vi "ReadRingConstant.vi"(1 "reference":refnum<vi>) -> (0 "RingConstant":T6)   [LabVIEW 2013]
uses:
  <vilib>/Utility/miscctls.llb/LVBoundsTypeDef.ctl
  <vilib>/Utility/miscctls.llb/LVPositionTypeDef.ctl
  <vilib>/Utility/miscctls.llb/LVRectTypeDef.ctl
  <vilib>/numeric/LVNumericRepresentation.ctl
  <vilib>/Utility/miscctls.llb/LVStringsAndValuesArrayTypeDef.ctl
panel:
  out "error out 29":errorcluster
  out "error out 28":errorcluster
  out "error out 27":errorcluster
  out "error out 26":errorcluster
  out "error out 25":errorcluster
  out "error out 24":errorcluster
  out "error out 23":errorcluster
  out "error out 22":errorcluster
  out "error out 21":errorcluster
  out "error out 20":errorcluster
  out "error out 19":errorcluster
  out "error out 18":errorcluster
  out "error out 17":errorcluster
  out "error out 16":errorcluster
  out "error out 15":errorcluster
  out "error out 14":errorcluster
  out "error out 13":errorcluster
  out "error out 12":errorcluster
  out "error out 11":errorcluster
  out "error out 10":errorcluster
  out "error out 9":errorcluster
  out "error out 8":errorcluster
  out "error out 7":errorcluster
  out "error out 6":errorcluster
  out "error out 5":errorcluster
  out "error out 4":errorcluster
  out "error out 3":errorcluster
  out "error out 2":errorcluster
  out "error out":errorcluster
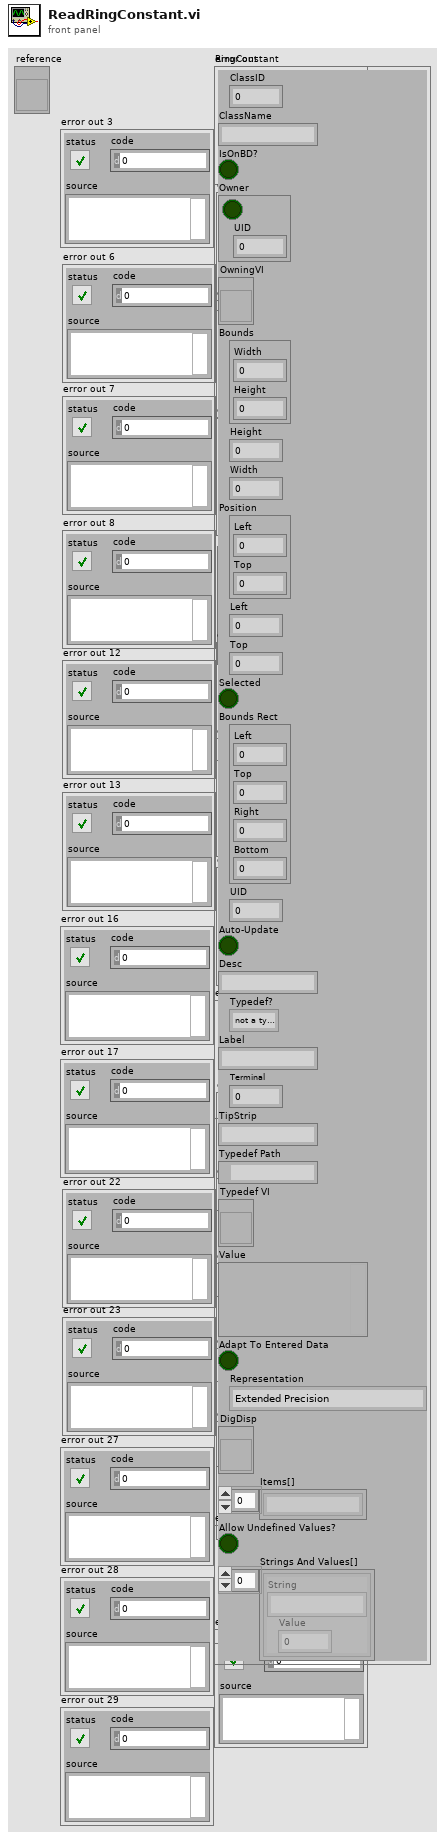
[diagram p1: front panel]
types:
  T1 = typedef "LVBoundsTypeDef.ctl" = cluster{"Width":u32, "Height":u32}
  T2 = typedef "LVPositionTypeDef.ctl" = cluster{"Left":i32, "Top":i32}
  T3 = typedef "LVRectTypeDef.ctl" = cluster{"Left":i16, "Top":i16, "Right":i16, "Bottom":i16}
  T4 = typedef "LVNumericRepresentation.ctl" = enum32{"Extended Precision", "Double Precision", "Single Precision", "Long", "Word", "Byte", "Unsigned Long", "Unsigned Word", "Unsigned Byte", "Complex Extended", "Complex Double", "Complex Single", "Quad", "Unsigned Quad", "Fixed-Point"}
  T5 = typedef "LVStringsAndValuesArrayTypeDef.ctl" = cluster{"String":string, "Value":ext}[]
  T6 = cluster{"ClassID":u32, "ClassName":string, "IsOnBD?":bool, "Owner":cluster{bool, "UID":i32}, "OwningVI":refnum<vi>, "Bounds":T1, "Height":u32, "Width":u32, "Position":T2, "Left":i32, "Top":i32, "Selected":bool, "Bounds Rect":T3, "UID":i32, "Auto-Update":bool, "Desc":string, "Typedef?":enum32{"not a typedef", "typedef", "strict typedef", "class private data"}, "Label":string, "Terminal":i32, "TipStrip":string, "Typedef Path":path, "Typedef VI":refnum<vi>, "Value":variant, "Adapt To Entered Data":bool, "Representation":T4, "DigDisp":refnum<vi>, "Items[]":string[], "Allow Undefined Values?":bool, "Strings And Values[]":T5}
  T7 = enum32{"not a typedef", "typedef", "strict typedef", "class private data"}
  T8 = cluster{"ClassID":u32, "ClassName":string, "IsOnBD?":bool, "Cluster":cluster{bool, "UID":i32}, "OwningVI":refnum<vi>, "Bounds":T1, "Height":u32, "Width":u32, "Position":T2, "Left":i32, "Top":i32, "Selected":bool, "Bounds Rect":T3, "UID":i32, "Auto-Update":bool, "Desc":string, "Typedef?":enum32{"not a typedef", "typedef", "strict typedef", "class private data"}, "Text":string, "UID":i32, "TipStrip":string, "Typedef Path":path, "Typedef VI":refnum<vi>, "Value":variant, "Adapt To Entered Data":bool, "Representation":T4, "DigDisp":refnum<vi>, "Items[]":string[], "Allow Undefined Values?":bool, "Strings And Values[]":T5}
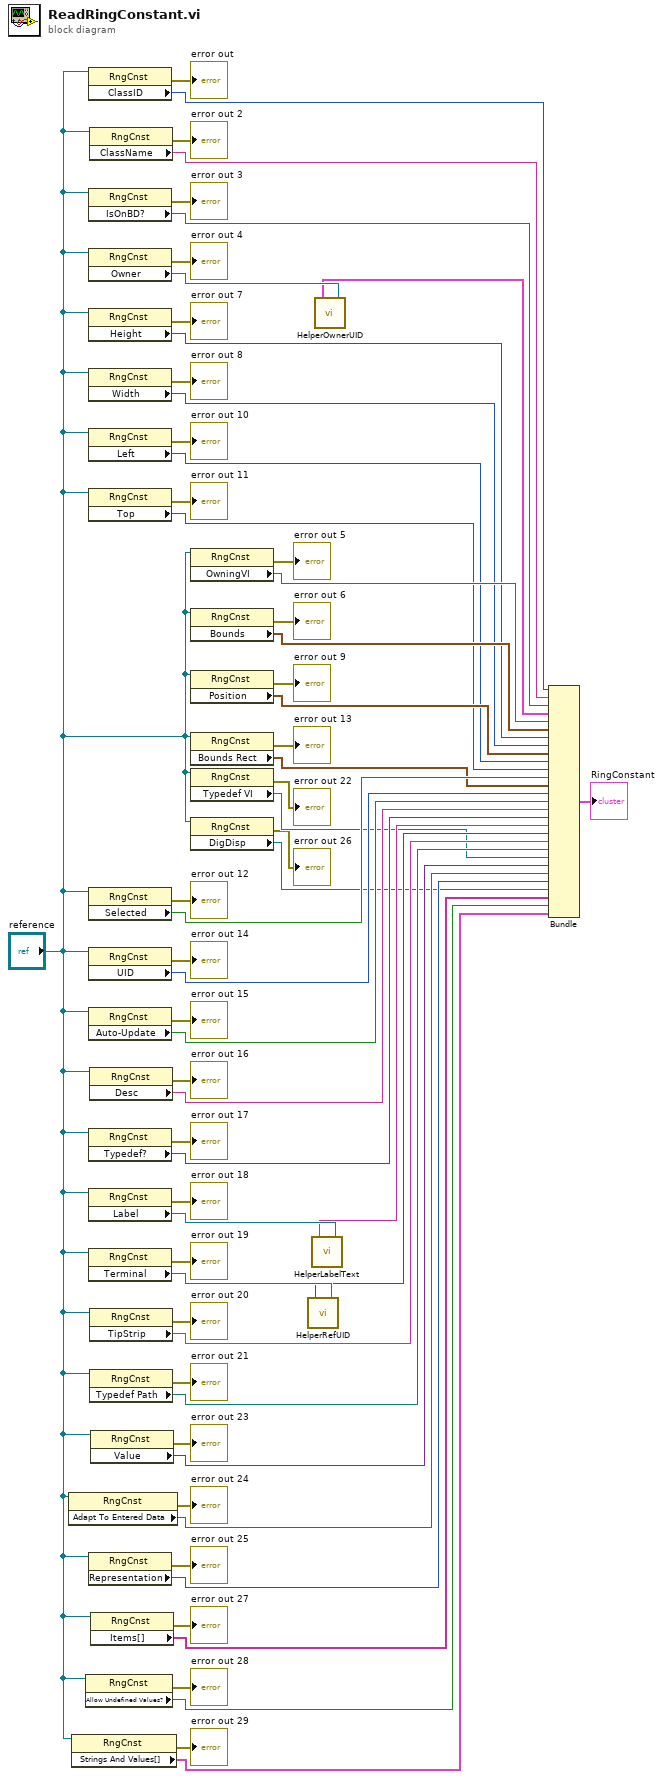
[diagram p0: block diagram]
diagram:
  n1 = property class="RngCnst"(reference="reference") -> (error out=→"error out 24":errorcluster, "Adapt To Entered Data"=w12:bool)  [unwired: 1 in, 1 out]
  n2 = property class="RngCnst"(reference="reference") -> (error out=→"error out 29":errorcluster, "Strings And Values[]"=w2:T5)  [unwired: 1 in, 1 out]
  n3 = property class="RngCnst"(reference="reference") -> (error out=→"error out 28":errorcluster, "Allow Undefined Values?"=w4:bool)  [unwired: 1 in, 1 out]
  n4 = property class="RngCnst"(reference="reference") -> (error out=→"error out":errorcluster, "ClassID"=w61:u32)  [unwired: 1 in, 1 out]
  n5 = property class="RngCnst"(reference="reference") -> (error out=→"error out 3":errorcluster, "IsOnBD?"=w57:bool)  [unwired: 1 in, 1 out]
  n6 = property class="RngCnst"(reference="reference") -> (error out=→"error out 4":errorcluster, "Owner"=w55:refnum<vi>)  [unwired: 1 in, 1 out]
  n7 = property class="RngCnst"(reference="reference") -> (error out=→"error out 7":errorcluster, "Height"=w48:u32)  [unwired: 1 in, 1 out]
  n8 = property class="RngCnst"(reference="reference") -> (error out=→"error out 8":errorcluster, "Width"=w46:u32)  [unwired: 1 in, 1 out]
  n9 = property class="RngCnst"(reference="reference") -> (error out=→"error out 10":errorcluster, "Left"=w42:i32)  [unwired: 1 in, 1 out]
  n10 = property class="RngCnst"(reference="reference") -> (error out=→"error out 11":errorcluster, "Top"=w40:i32)  [unwired: 1 in, 1 out]
  n11 = property class="RngCnst"(reference="reference") -> (error out=→"error out 12":errorcluster, "Selected"=w38:bool)  [unwired: 1 in, 1 out]
  n12 = property class="RngCnst"(reference="reference") -> (error out=→"error out 14":errorcluster, "UID"=w34:i32)  [unwired: 1 in, 1 out]
  n13 = property class="RngCnst"(reference="reference") -> (error out=→"error out 15":errorcluster, "Auto-Update"=w32:bool)  [unwired: 1 in, 1 out]
  n14 = property class="RngCnst"(reference="reference") -> (error out=→"error out 17":errorcluster, "Typedef?"=w28:T7)  [unwired: 1 in, 1 out]
  n15 = property class="RngCnst"(reference="reference") -> (error out=→"error out 18":errorcluster, "Label"=w26:refnum<vi>)  [unwired: 1 in, 1 out]
  n16 = property class="RngCnst"(reference="reference") -> (error out=→"error out 19":errorcluster, "Terminal"=w23:refnum<vi>)  [unwired: 1 in, 1 out]
  n17 = property class="RngCnst"(reference="reference") -> (error out=→"error out 25":errorcluster, "Representation"=w10:T4)  [unwired: 1 in, 1 out]
  n18 = property class="RngCnst"(reference="reference") -> (error out=→"error out 2":errorcluster, "ClassName"=w59:string)  [unwired: 1 in, 1 out]
  n19 = property class="RngCnst"(reference="reference") -> (error out=→"error out 16":errorcluster, "Desc"=w30:string)  [unwired: 1 in, 1 out]
  n20 = property class="RngCnst"(reference="reference") -> (error out=→"error out 20":errorcluster, "TipStrip"=w20:string)  [unwired: 1 in, 1 out]
  n21 = property class="RngCnst"(reference="reference") -> (error out=→"error out 21":errorcluster, "Typedef Path"=w18:path)  [unwired: 1 in, 1 out]
  n22 = property class="RngCnst"(reference="reference") -> (error out=→"error out 23":errorcluster, "Value"=w14:variant)  [unwired: 1 in, 1 out]
  n23 = property class="RngCnst"(reference="reference") -> (error out=→"error out 27":errorcluster, "Items[]"=w6:string[])  [unwired: 1 in, 1 out]
  n24 = property class="RngCnst"(reference="reference") -> (error out=→"error out 5":errorcluster, "OwningVI"=w52:refnum<vi>)  [unwired: 1 in, 1 out]
  n25 = property class="RngCnst"(reference="reference") -> (error out=→"error out 6":errorcluster, "Bounds"=w50:T1)  [unwired: 1 in, 1 out]
  n26 = property class="RngCnst"(reference="reference") -> (error out=→"error out 9":errorcluster, "Position"=w44:T2)  [unwired: 1 in, 1 out]
  n27 = property class="RngCnst"(reference="reference") -> (error out=→"error out 13":errorcluster, "Bounds Rect"=w36:T3)  [unwired: 1 in, 1 out]
  n28 = property class="RngCnst"(reference="reference") -> (error out=→"error out 22":errorcluster, "Typedef VI"=w16:refnum<vi>)  [unwired: 1 in, 1 out]
  n29 = property class="RngCnst"(reference="reference") -> (error out=→"error out 26":errorcluster, "DigDisp"=w8:refnum<vi>)  [unwired: 1 in, 1 out]
  n30 = call "HelperRefUID.vi"("Text in"=w23) -> ("UID"=w22:i32)
  n31 = call "HelperLabelText.vi"("Text in"=w26) -> ("Text"=w25:string)
  n32 = call "HelperOwnerUID.vi"("Generic in"=w55) -> ("Cluster"=w54:cluster{bool, "UID":i32})
  n33 = Bundle("ClassID"=w61, "ClassName"=w59, "IsOnBD?"=w57, "Cluster"=w54, "OwningVI"=w52, "Bounds"=w50, "Height"=w48, "Width"=w46, "Position"=w44, "Left"=w42, "Top"=w40, "Selected"=w38, "Bounds Rect"=w36, "UID"=w34, "Auto-Update"=w32, "Desc"=w30, "Typedef?"=w28, "Text"=w25, "UID"=w22, "TipStrip"=w20, "Typedef Path"=w18, "Typedef VI"=w16, "Value"=w14, "Adapt To Entered Data"=w12, "Representation"=w10, "DigDisp"=w8, "Items[]"=w6, "Allow Undefined Values?"=w4, "Strings And Values[]"=w2) -> (→"RingConstant":T8)  [unwired: 1 in]
